vi "Configure Measurement (Channel Power Filter).vi"(0 "VISA resource name":refnum<visa-resource-name>, 1 "RRC Filter Bandwidth (2E+6 Hz)":dbl=2000000.0, 5 "Enable RRC Filter (F: Disable)":bool, 9 "RRC Filter Alpha Value (1)":dbl=1.0, 11 "error in (no error)":errorcluster) -> (4 "VISA resource name out":refnum<visa-resource-name>, 15 "error out":errorcluster)   [LabVIEW 2022 SP3, in "Agilent N934X Series.lvlib"]
doc: "Configures the filter settings of Channel Power measurement type.\n\nNote:\nThis VI is only applicable for N9321C, N9322C, N9323C, N9324C."
uses:
  <instrlib>/Agilent N934X Series/Agilent N934X Series.lvlib
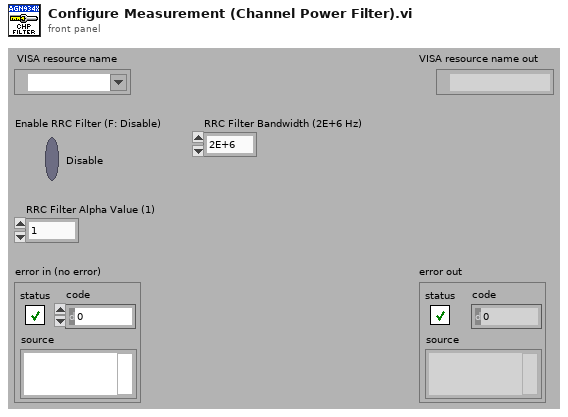
[diagram p1: front panel]
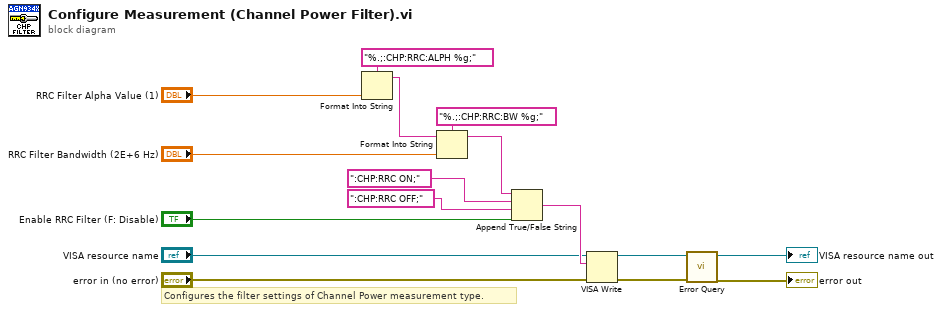
[diagram p0: block diagram]
diagram:
  # "Configures the filter settings of Channel Power measurement type."
  n1 = Format Into String(format string="%.;:CHP:RRC:ALPH %g;", "RRC Filter Alpha Value (1)") -> (resulting string=w1:string)  [unwired: 2 in, 1 out]
  n2 = Format Into String(format string="%.;:CHP:RRC:BW %g;", initial string=w1, "RRC Filter Bandwidth (2E+6 Hz)") -> (resulting string=w12:string)  [unwired: 1 in, 1 out]
  n3 = Append True/False String(1:"Enable RRC Filter (F: Disable)", 2:":CHP:RRC OFF;", 3:":CHP:RRC ON;", 4:w12) -> (0:w8:string)
  n4 = VISA Write(VISA resource name="VISA resource name", write buffer=w8, error in (no error)="error in (no error)") -> (VISA resource name out=w5:refnum<visa-resource-name>, error out=w4:errorcluster)  [unwired: 1 out]
  n5 = call <instrlib>:"Error Query.vi"("error in (no error)"=w4, "VISA resource name"=w5) -> ("error out"=→"error out":errorcluster, "VISA resource name out"=→"VISA resource name out":refnum<visa-resource-name>)  [unwired: 6 in, 2 out]
